vi "FastBeamMode.vi"() -> ()   [LabVIEW 2021]
uses:
  D:/tmytek/Source/bbox-api/example/BBoxOne Series/LabVIEW/BBoxAPI.dll
  BBoxAPI.dll
  kernel32.dll
panel:
  out "getAAKitList":string[](array[string])
  out "Exists Table Filenames":string[](array[string])
  out "Get Current Working Directory":path
  in  "Set Current Working Directory":path
  out "SN":string
  out "Init":i32(ring)=13 items=["OK"=0, "WARNING"=1, "ERROR"=2, "NO_RESPONSE"=3, "ERROR_GET_SN"=10, "ERROR_DEV_TYPE"=11, "ERROR_INIT_OBJECT"=12, "ERROR_DEV_NOT_INIT"=13, "ERROR_METHOD_NOT_FOUND"=14, "ERROR_REFLECTION"=15, "ERROR_POWER"=16, "ERROR_NETWORK_NOT_INIT"=20, "ERROR_NETWORK_INIT"=21, "ERROR_NETWORK_CONNECT_TIMEOUT"=22, "ERROR_DISCONNECT"=23, "ERROR_SOCKET"=24, "ERROR_SEND_CMD"=25, "ERROR_RESP_CMD"=26, "ERROR_DEV_COUNT_ZERO"=30, "ERROR_CMD"=40, "ERROR_CMD_INIT"=41, "ERROR_BF_AAKIT"=100, "ERROR_BF_NO_AAKIT"=101, "ERROR_BF_CALI_PATH"=102, "ERROR_BF_BEAMXY"=103, "ERROR_BF_GEN"=104, "ERROR_BF_TRMODE"=105, "STATUS_BF_LOAD_CALI_INCOMPLTE"=106, "ERROR_BF_LOAD_CALI_PARSE_FAILED"=107, "ERROR_FREQ_EQUATION"=250, "ERROR_PLO_CRC"=251, "WARNING_HARMONIC"=252, "ERROR_HARMONIC_BLOCK"=253]
  out "getFrequencyList":string[](array[string])
  out "setOperatingFreq":i32(ring)=13 items=["OK"=0, "WARNING"=1, "ERROR"=2, "NO_RESPONSE"=3, "ERROR_GET_SN"=10, "ERROR_DEV_TYPE"=11, "ERROR_INIT_OBJECT"=12, "ERROR_DEV_NOT_INIT"=13, "ERROR_METHOD_NOT_FOUND"=14, "ERROR_REFLECTION"=15, "ERROR_POWER"=16, "ERROR_NETWORK_NOT_INIT"=20, "ERROR_NETWORK_INIT"=21, "ERROR_NETWORK_CONNECT_TIMEOUT"=22, "ERROR_DISCONNECT"=23, "ERROR_SOCKET"=24, "ERROR_SEND_CMD"=25, "ERROR_RESP_CMD"=26, "ERROR_DEV_COUNT_ZERO"=30, "ERROR_CMD"=40, "ERROR_CMD_INIT"=41, "ERROR_BF_AAKIT"=100, "ERROR_BF_NO_AAKIT"=101, "ERROR_BF_CALI_PATH"=102, "ERROR_BF_BEAMXY"=103, "ERROR_BF_GEN"=104, "ERROR_BF_TRMODE"=105, "STATUS_BF_LOAD_CALI_INCOMPLTE"=106, "ERROR_BF_LOAD_CALI_PARSE_FAILED"=107, "ERROR_FREQ_EQUATION"=250, "ERROR_PLO_CRC"=251, "WARNING_HARMONIC"=252, "ERROR_HARMONIC_BLOCK"=253]
  out "selectAAKit":i32(ring)=13 items=["OK"=0, "WARNING"=1, "ERROR"=2, "NO_RESPONSE"=3, "ERROR_GET_SN"=10, "ERROR_DEV_TYPE"=11, "ERROR_INIT_OBJECT"=12, "ERROR_DEV_NOT_INIT"=13, "ERROR_METHOD_NOT_FOUND"=14, "ERROR_REFLECTION"=15, "ERROR_POWER"=16, "ERROR_NETWORK_NOT_INIT"=20, "ERROR_NETWORK_INIT"=21, "ERROR_NETWORK_CONNECT_TIMEOUT"=22, "ERROR_DISCONNECT"=23, "ERROR_SOCKET"=24, "ERROR_SEND_CMD"=25, "ERROR_RESP_CMD"=26, "ERROR_DEV_COUNT_ZERO"=30, "ERROR_CMD"=40, "ERROR_CMD_INIT"=41, "ERROR_BF_AAKIT"=100, "ERROR_BF_NO_AAKIT"=101, "ERROR_BF_CALI_PATH"=102, "ERROR_BF_BEAMXY"=103, "ERROR_BF_GEN"=104, "ERROR_BF_TRMODE"=105, "STATUS_BF_LOAD_CALI_INCOMPLTE"=106, "ERROR_BF_LOAD_CALI_PARSE_FAILED"=107, "ERROR_FREQ_EQUATION"=250, "ERROR_PLO_CRC"=251, "WARNING_HARMONIC"=252, "ERROR_HARMONIC_BLOCK"=253]
  in  "Target Freq Index":i32 min=1 max=2 step=1
  in  "Target AAKit Index":i32 min=1 max=2 step=1
  out "Target AAKit Name":string
  in  "Fast BeamMode Enable":bool=TRUE
  out "Set_Fast_Parallel_Mode":i32(ring) items=["OK"=0, "WARNING"=1, "ERROR"=2, "NO_RESPONSE"=3, "ERROR_GET_SN"=10, "ERROR_DEV_TYPE"=11, "ERROR_INIT_OBJECT"=12, "ERROR_DEV_NOT_INIT"=13, "ERROR_METHOD_NOT_FOUND"=14, "ERROR_REFLECTION"=15, "ERROR_POWER"=16, "ERROR_SCAN_NOT_FOUND"=17, "ERROR_UNMATCH_RETURN_TYPE"=18, "ERROR_NETWORK_NOT_INIT"=20, "ERROR_NETWORK_INIT"=21, "ERROR_NETWORK_CONNECT_TIMEOUT"=22, "ERROR_DISCONNECT"=23, "ERROR_SOCKET"=24, "ERROR_SEND_CMD"=25, "ERROR_RESP_CMD"=26, "ERROR_DEV_COUNT_ZERO"=30, "ERROR_DEV_DUMMY_FUNC"=31, "ERROR_CMD"=40, "ERROR_CMD_INIT"=41, "ERROR_BF_AAKIT"=100, "ERROR_BF_NO_AAKIT"=101, "ERROR_BF_CALI_PATH"=102, "ERROR_BF_BEAMXY"=103, "ERROR_BF_GEN"=104, "ERROR_BF_TRMODE"=105, "STATUS_BF_LOAD_CALI_INCOMPLTE"=106, "ERROR_BF_LOAD_CALI_PARSE_FAILED"=107, "ERROR_BF_UNLOAD_CALI"=108, "ERROR_BF_CALI_VERSION_UNSUPPORTED"=109, "ERROR_BF_CALI_DATA_NOT_FOUND"=110, "ERROR_FREQ_EQUATION"=250, "ERROR_PLO_CRC"=251, "WARNING_HARMONIC"=252, "ERROR_HARMONIC_BLOCK"=253, "ERROR_FW_UPGRADE_IP_INVALID"=300, "ERROR_FW_VERSION_NOT_SUPPORT"=301]
  out "ScanningDevice":string[](array[string])
  # "Notice:\n\nThe Set / Get Current Working Diectory Path must be \nthe sample code directory path\n\nbbox-api\\example\\BBoxOne Series\\LabVIEW\\\n\nand must exist\n\nbbox-api\\example\\BBoxOne Series\\LabVIEW\\BBoxAPI.dll\n\nbbox-api\\example\\BBoxOne Series\\LabVIEW\\files\\\n\nbbox-api\\example\\BBoxOne Series\\LabVIEW\\logs\\"
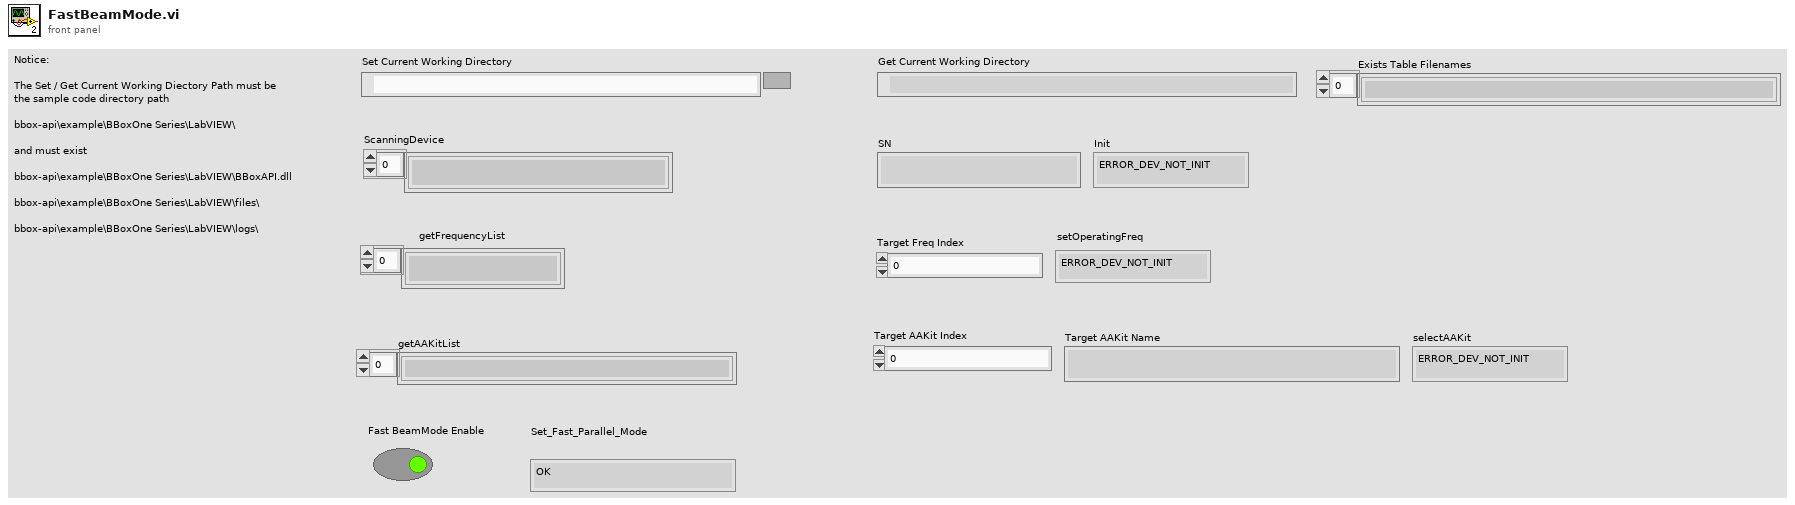
[diagram p1: front panel]
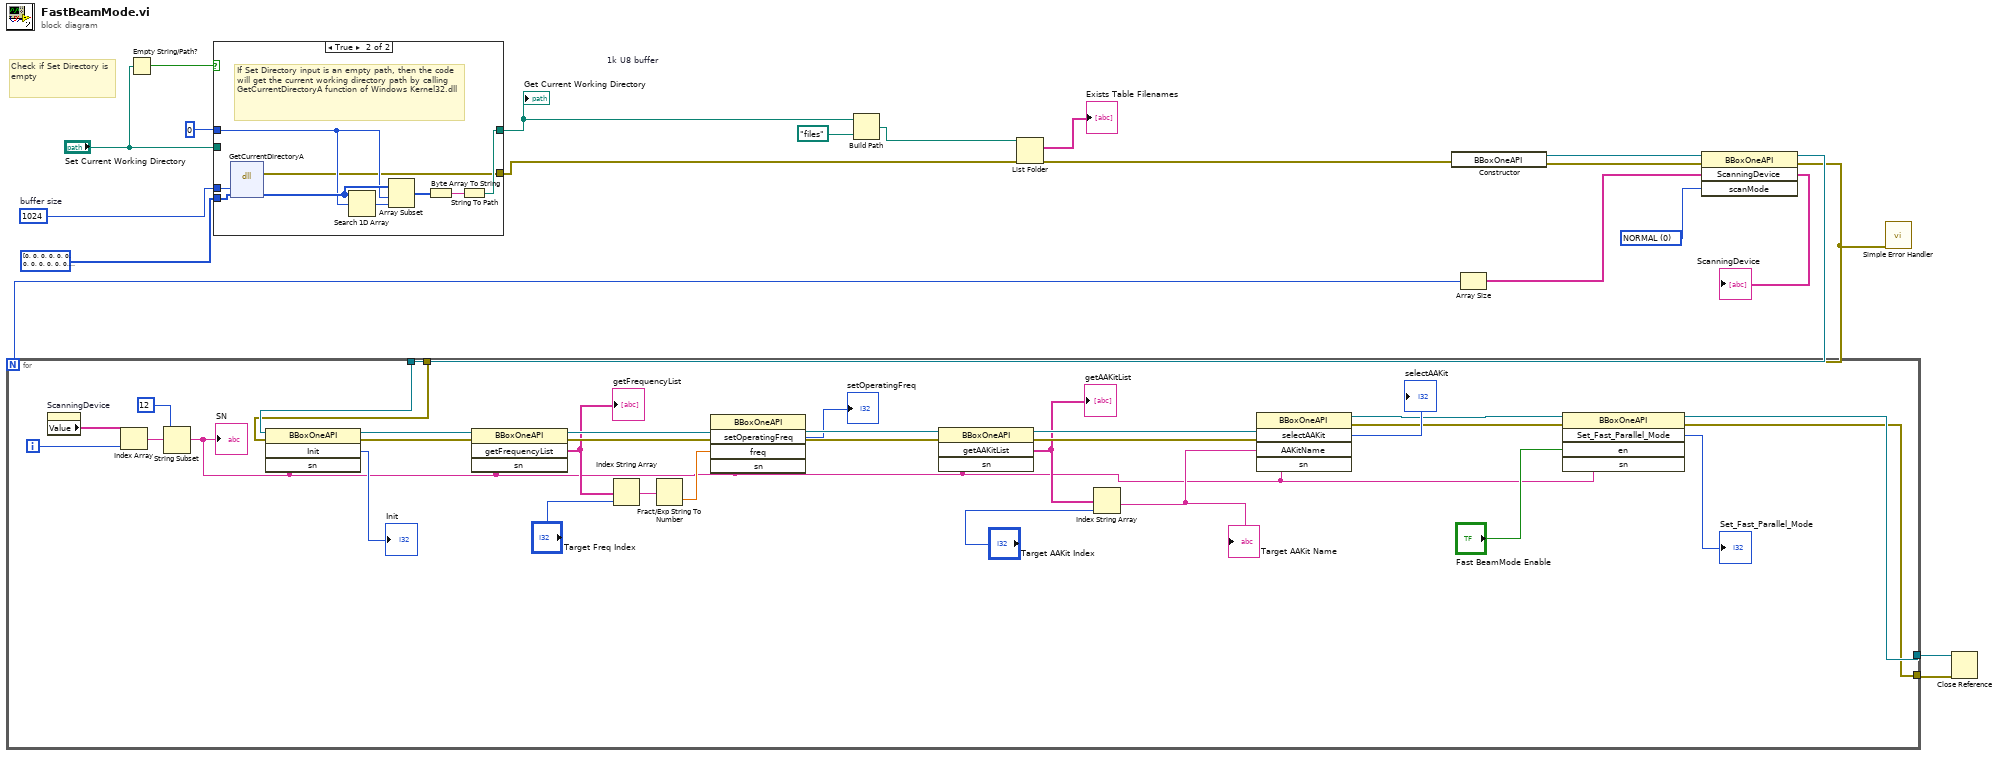
[diagram p0: block diagram]
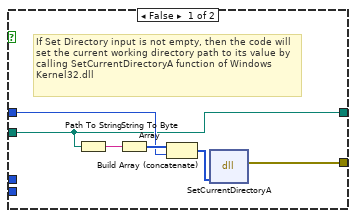
[diagram p2: hidden frame]
diagram:
  w9 = 1024  # buffer size
  w8 = u8[] [0, 0, 0, 0, 0, 0, 0, 0, 0, 0, 0, 0, 0, 0, 0, 0, 0, 0, 0, 0, 0, 0, 0, 0, 0, 0, 0, 0, 0, 0, 0, 0, 0, 0, 0, 0, 0, 0, 0, 0, 0, 0, 0, 0, 0, 0, 0, 0, 0, 0, 0, 0, 0, 0, 0, 0, 0, 0, 0, 0, 0, 0, 0, 0, 0, 0, 0, 0, 0, 0, 0, 0, 0, 0, 0, 0, 0, 0, 0, 0, 0, 0, 0, 0, 0, 0, 0, 0, 0, 0, 0, 0, 0, 0, 0, 0, 0, 0, 0, 0, 0, 0, 0, 0, 0, 0, 0, 0, 0, 0, 0, 0, 0, 0, 0, 0, 0, 0, 0, 0, 0, 0, 0, 0, 0, 0, 0, 0, 0, 0, 0, 0, 0, 0, 0, 0, 0, 0, 0, 0, 0, 0, 0, 0, 0, 0, 0, 0, 0, 0, 0, 0, 0, 0, 0, 0, 0, 0, 0, 0, 0, 0, 0, 0, 0, 0, 0, 0, 0, 0, 0, 0, 0, 0, 0, 0, 0, 0, 0, 0, 0, 0, 0, 0, 0, 0, 0, 0, 0, 0, 0, 0, 0, 0, 0, 0, 0, 0, 0, 0, 0, 0, 0, 0, 0, 0, 0, 0, 0, 0, 0, 0, 0, 0, 0, 0, 0, 0, 0, 0, 0, 0, 0, 0, 0, 0, 0, 0, 0, 0, 0, 0, 0, 0, 0, 0, 0, 0, 0, 0, 0, 0, 0, 0, 0, 0, 0, 0, 0, 0, 0, 0, 0, 0, 0, 0, 0, 0, 0, 0, 0, 0, 0, 0, 0, 0, 0, 0, 0, 0, 0, 0, 0, 0, 0, 0, 0, 0, 0, 0, 0, 0, 0, 0, 0, 0, 0, 0, 0, 0, 0, 0, 0, 0, 0, 0, 0, 0, 0, 0, 0, 0, 0, 0, 0, 0, 0, 0, 0, 0, 0, 0, 0, 0, 0, 0, 0, 0, 0, 0, 0, 0, 0, 0, 0, 0, 0, 0, 0, 0, 0, 0, 0, 0, 0, 0, 0, 0, 0, 0, 0, 0, 0, 0, 0, 0, 0, 0, 0, 0, 0, 0, 0, 0, 0, 0, 0, 0, 0, 0, 0, 0, 0, 0, 0, 0, 0, 0, 0, 0, 0, 0, 0, 0, 0, 0, 0, 0, 0, 0, 0, 0, 0, 0, 0, 0, 0, 0, 0, 0, 0, 0, 0, 0, 0, 0, 0, 0, 0, 0, 0, 0, 0, 0, 0, 0, 0, 0, 0, 0, 0, 0, 0, 0, 0, 0, 0, 0, 0, 0, 0, 0, 0, 0, 0, 0, 0, 0, 0, 0, 0, 0, 0, 0, 0, 0, 0, 0, 0, 0, 0, 0, 0, 0, 0, 0, 0, 0, 0, 0, 0, 0, 0, 0, 0, 0, 0, 0, 0, 0, 0, 0, 0, 0, 0, 0, 0, 0, 0, 0, 0, 0, 0, 0, 0, 0, 0, 0, 0, 0, 0, 0, 0, 0, 0, 0, 0, 0, 0, 0, 0, 0, 0, 0, 0, 0, 0, 0, 0, 0, 0, 0, 0, 0, 0, 0, 0, 0, 0, 0, 0, 0, 0, 0, 0, 0, 0, 0, 0, 0, 0, 0, 0, 0, 0, 0, 0, 0, 0, 0, 0, 0, 0, 0, 0, 0, 0, 0, 0, 0, 0, 0, 0, 0, 0, 0, 0, 0, 0, 0, 0, 0, 0, 0, 0, 0, 0, 0, 0, 0, 0, 0, 0, 0, 0, 0, 0, 0, 0, 0, 0, 0, 0, 0, 0, 0, 0, 0, 0, 0, 0, 0, 0, 0, 0, 0, 0, 0, 0, 0, 0, 0, 0, 0, 0, 0, 0, 0, 0, 0, 0, 0, 0, 0, 0, 0, 0, 0, 0, 0, 0, 0, 0, 0, 0, 0, 0, 0, 0, 0, 0, 0, 0, 0, 0, 0, 0, 0, 0, 0, 0, 0, 0, 0, 0, 0, 0, 0, 0, 0, 0, 0, 0, 0, 0, 0, 0, 0, 0, 0, 0, 0, 0, 0, 0, 0, 0, 0, 0, 0, 0, 0, 0, 0, 0, 0, 0, 0, 0, 0, 0, 0, 0, 0, 0, 0, 0, 0, 0, 0, 0, 0, 0, 0, 0, 0, 0, 0, 0, 0, 0, 0, 0, 0, 0, 0, 0, 0, 0, 0, 0, 0, 0, 0, 0, 0, 0, 0, 0, 0, 0, 0, 0, 0, 0, 0, 0, 0, 0, 0, 0, 0, 0, 0, 0, 0, 0, 0, 0, 0, 0, 0, 0, 0, 0, 0, 0, 0, 0, 0, 0, 0, 0, 0, 0, 0, 0, 0, 0, 0, 0, 0, 0, 0, 0, 0, 0, 0, 0, 0, 0, 0, 0, 0, 0, 0, 0, 0, 0, 0, 0, 0, 0, 0, 0, 0, 0, 0, 0, 0, 0, 0, 0, 0, 0, 0, 0, 0, 0, 0, 0, 0, 0, 0, 0, 0, 0, 0, 0, 0, 0, 0, 0, 0, 0, 0, 0, 0, 0, 0, 0, 0, 0, 0, 0, 0, 0, 0, 0, 0, 0, 0, 0, 0, 0, 0, 0, 0, 0, 0, 0, 0, 0, 0, 0, 0, 0, 0, 0, 0, 0, 0, 0, 0, 0, 0, 0, 0, 0, 0, 0, 0, 0, 0, 0, 0, 0, 0, 0, 0, 0, 0, 0, 0, 0, 0, 0, 0, 0, 0, 0, 0, 0, 0, 0, 0, 0, 0, 0, 0, 0, 0, 0, 0, 0, 0, 0, 0, 0, 0, 0, 0, 0, 0, 0, 0, 0, 0, 0, 0, 0, 0, 0, 0, 0, 0, 0, 0, 0, 0, 0, 0, 0, 0, 0, 0, 0, 0, 0, 0, 0, 0, 0, 0, 0, 0, 0, 0, 0, 0, 0, 0, 0, 0, 0, 0, 0, 0, 0, 0, 0, 0, 0, 0, 0, 0, 0, 0, 0, 0, 0, 0, 0, 0, 0, 0, 0, 0, 0, 0, 0, 0, 0, 0, 0, 0, 0, 0, 0, 0, 0, 0, 0, 0, 0, 0, 0, 0, 0, 0, 0, 0, 0, 0, 0, 0, 0, 0, 0, 0, 0, 0, 0, 0, 0, 0, 0, 0, 0, 0, 0, 0, 0, 0, 0, 0, 0, 0, 0, 0, 0, 0, 0, 0, 0, 0, 0, 0, 0, 0, 0, 0, 0, 0]  # 1k U8 buffer
  w20 = 0 items=["NORMAL", "FAST"] ("scanMode")
  # "Check if Set Directory is empty"
  n1 = Empty String/Path?(string/path="Set Current Working Directory") -> (empty?=w10:bool)
  n2 = case shown="True" w10 {
    tunnel: "Set Current Working Directory" -> [w22 _]
    tunnel: u8 0 -> [w24 w31]
    tunnel: w9 -> [_ w30]
    tunnel: w8 -> [_ w29]
    tunnel: [w22 w28] -> w3
    tunnel: [w21 w27] -> w2
    frame False {
      # "If Set Directory input is not empty, then the code will set the current working directory path to its value by calling SetCurrentDirectoryA function of Windows Kernel32.dll"
      n3 = Path To String(path=w22) -> (string=w23:string)
      n4 = String To Byte Array(string=w23) -> (unsigned byte array=w26:u8[])
      n5 = Build Array (concatenate)(w26, w24) -> (w25:u8[])
      n6 = dll-call lib="Kernel32.dll" fn="SetCurrentDirectoryA" label="Kernel32.dll - \nSetCurrentDirectoryA"("lpPathName"=w25) -> (error out=w21:errorcluster)  [unwired: 4 in, 2 out]
    }
    frame True {
      # "If Set Directory input is an empty path, then the code will get the current working directory path by calling GetCurrentDirectoryA function of Windows Kernel32.dll"
      n7 = dll-call lib="kernel32.dll" fn="GetCurrentDirectoryA" label="Kernel32.dll - \nGetCurrentDirectoryA"("nBufferLength"=w30, "lpBuffer"=w29) -> (error out=w27:errorcluster, "lpBuffer"=w34:u8[])  [unwired: 4 in, 2 out]
      n8 = Search 1D Array(1D array=w34, element=w31) -> (index of element=w35:i32)  [unwired: 1 out]
      n9 = Array Subset(array=w34, index=w31, length=w35) -> (w32:u8[])
      n10 = Byte Array To String(unsigned byte array=w32) -> (string=w33:string)
      n11 = String To Path(string=w33) -> (path=w28:path)
    }
  }
  "Get Current Working Directory" <- w3
  n12 = Build Path(base path=w3, name or relative path=path "files") -> (appended path=w4:path)
  n13 = List Folder(path=w4, error in=w2) -> (filenames=→"Exists Table Filenames":string[], error out=w1:errorcluster)  [unwired: 2 in, 2 out]
  n14 = constructor class="BBoxOneAPI"(error in=w1) -> (reference out=w19:refnum<k24>, error out=w18:errorcluster)  [unwired: 2 in, 1 out]
  n15 = invoke class="BBoxOneAPI" method="ScanningDevice"(reference=w19, error in=w18, "scanMode"=w20) -> (reference out=w15:refnum<k24>, error out=w14:errorcluster, "ScanningDevice"=w16:string[])  [unwired: 1 in, 1 out]
  "ScanningDevice" <- w16
  n16 = Array Size(array=w16) -> (size(s)=w17:i32)
  n17 = for {
    N: w17 -> [_]
    tunnel: w15 -> [w64]
    tunnel: w14 -> [w63]
    tunnel: [w37] -> w12
    tunnel: [w38] -> w13
    i -> [w51]
    n18 = property on="ScanningDevice" class="Arr (strict)"() -> ("Value"=w56:string[])  [unwired: 2 in, 2 out]
    n19 = Index Array(array=w56, index=w51) -> (element=w66:string)
    n20 = String Subset(string=w66, length (rest)=12) -> (substring=w36:string)  [unwired: 1 in]
    "SN" <- w36
    n21 = invoke class="BBoxOneAPI" method="Init"(reference=w64, error in=w63, "sn"=w36) -> (reference out=w55:refnum<k24>, error out=w54:errorcluster, "Init"=→"Init":i32)  [unwired: 1 in, 1 out]
    n22 = invoke class="BBoxOneAPI" method="getFrequencyList"(reference=w55, error in=w54, "sn"=w36) -> (reference out=w53:refnum<k24>, error out=w52:errorcluster, "getFrequencyList"=w49:string[])  [unwired: 1 in, 1 out]
    "getFrequencyList" <- w49
    n23 = Index String Array(1:"Target Freq Index", 2:w49) -> (0:w47:string)  [unwired: 1 in]
    n24 = Fract/Exp String To Number(string=w47) -> (number=w46:dbl)  [unwired: 3 in, 1 out]
    n25 = invoke class="BBoxOneAPI" method="setOperatingFreq"(reference=w53, error in=w52, "freq"=w46, "sn"=w36) -> (reference out=w60:refnum<k24>, error out=w59:errorcluster, "setOperatingFreq"=→"setOperatingFreq":i32)  [unwired: 1 in, 2 out]
    n26 = invoke class="BBoxOneAPI" method="getAAKitList"(reference=w60, error in=w59, "sn"=w36) -> (reference out=w58:refnum<k24>, error out=w57:errorcluster, "getAAKitList"=w45:string[])  [unwired: 1 in, 1 out]
    "getAAKitList" <- w45
    n27 = Index String Array(1:"Target AAKit Index", 2:w45) -> (0:w44:string)  [unwired: 1 in]
    "Target AAKit Name" <- w44
    n28 = invoke class="BBoxOneAPI" method="selectAAKit"(reference=w58, error in=w57, "AAKitName"=w44, "sn"=w36) -> (reference out=w41:refnum<k24>, error out=w40:errorcluster, "selectAAKit"=→"selectAAKit":i32)  [unwired: 1 in, 2 out]
    n29 = invoke class="BBoxOneAPI" method="Set_Fast_Parallel_Mode"(reference=w41, error in=w40, "en"="Fast BeamMode Enable", "sn"=w36) -> (reference out=w38:refnum<k24>, error out=w37:errorcluster, "Set_Fast_Parallel_Mode"=→"Set_Fast_Parallel_Mode":i32)  [unwired: 1 in, 2 out]
  }
  n30 = call <vilib>:"Simple Error Handler.vi"("error in (no error)"=w14) -> ()  [unwired: 4 in, 5 out]
  n31 = Close Reference(reference=w13, error in (no error)=w12) -> ()  [unwired: 1 out]
